vi "ETH 2 Main.vi"(7 "ETH2 Q":refnum<queue>, 8 "error in":errorcluster, 10 "connection ID":refnum<k5>, 11 "data in":string) -> (0 "error out":errorcluster, 2 "connection ID 2":refnum<k5>)   [LabVIEW 2022 SP3]
panel:
  in  "ETH2 Q 2":refnum<queue>
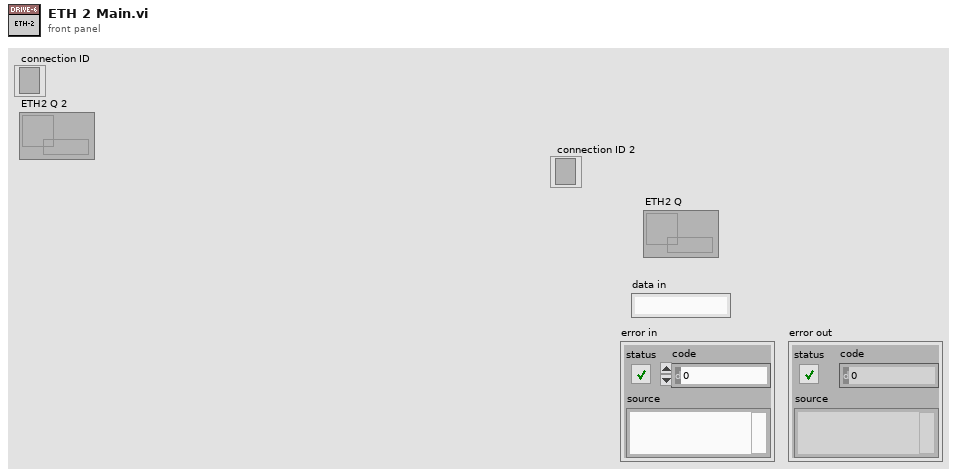
[diagram p1: front panel]
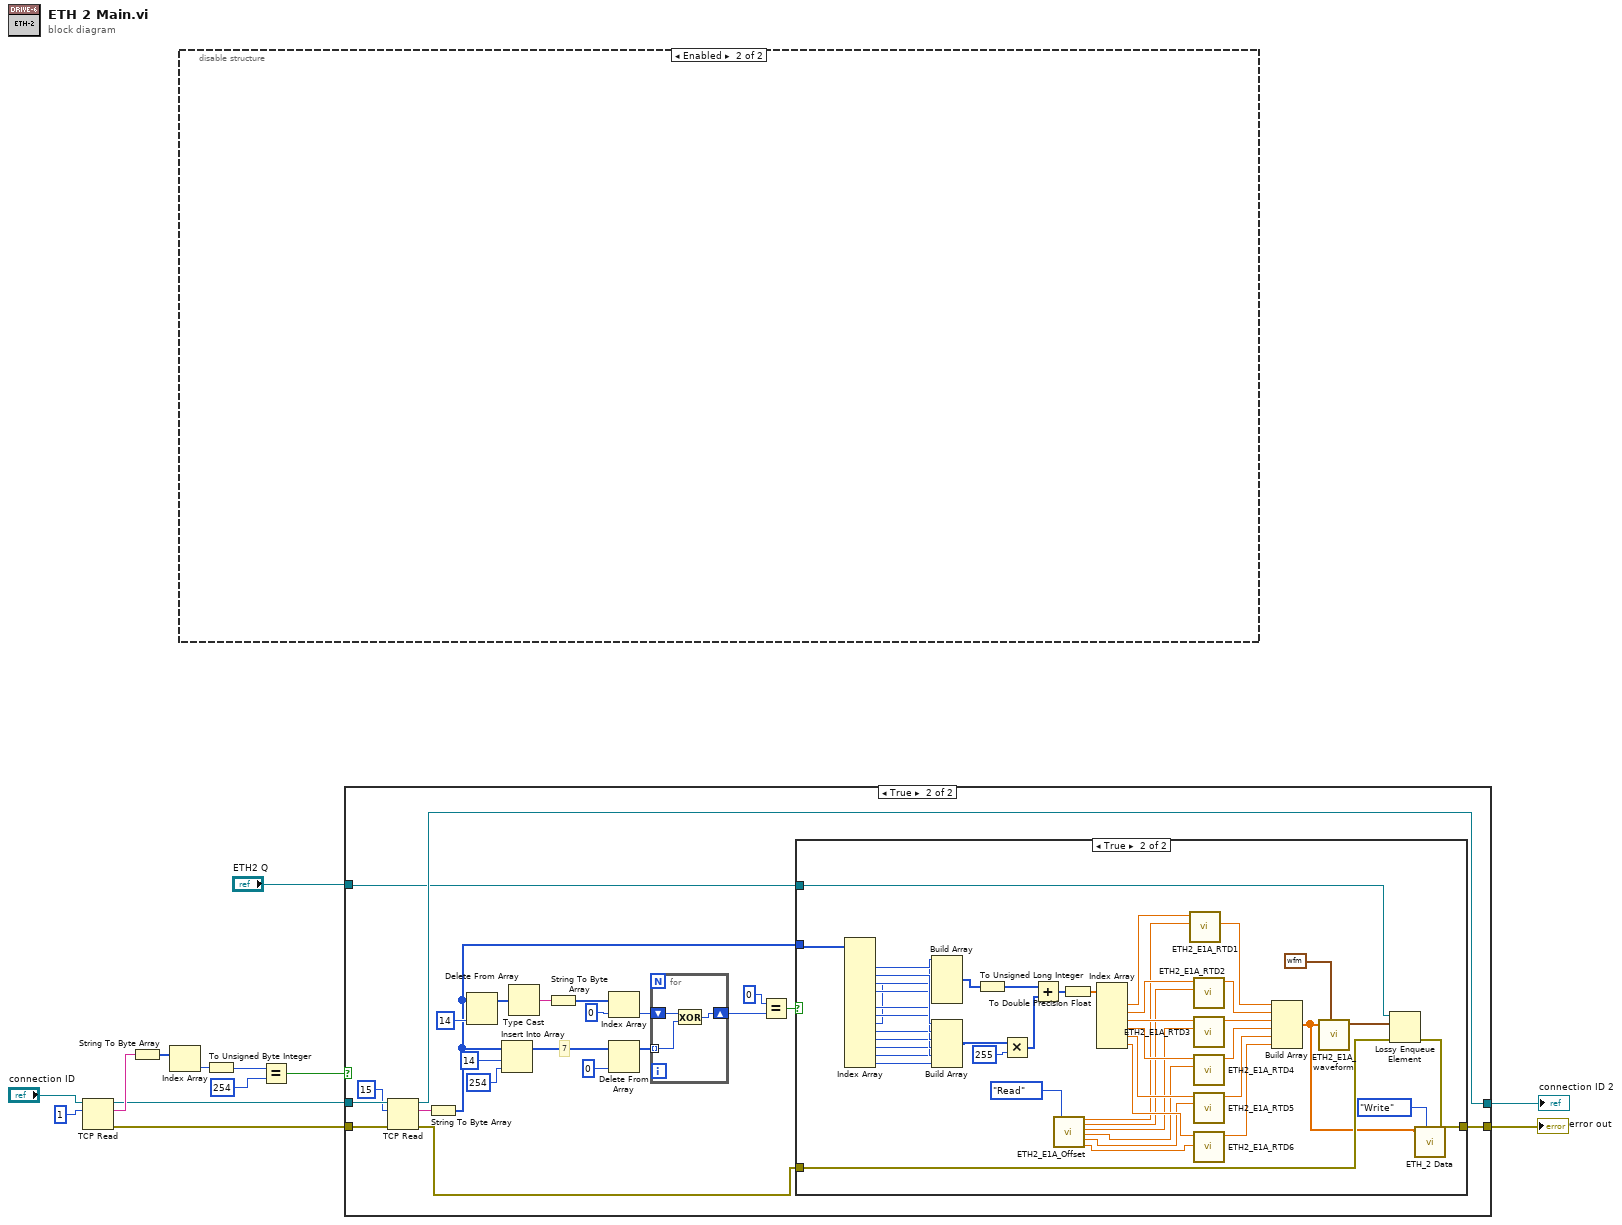
[diagram p0: block diagram]
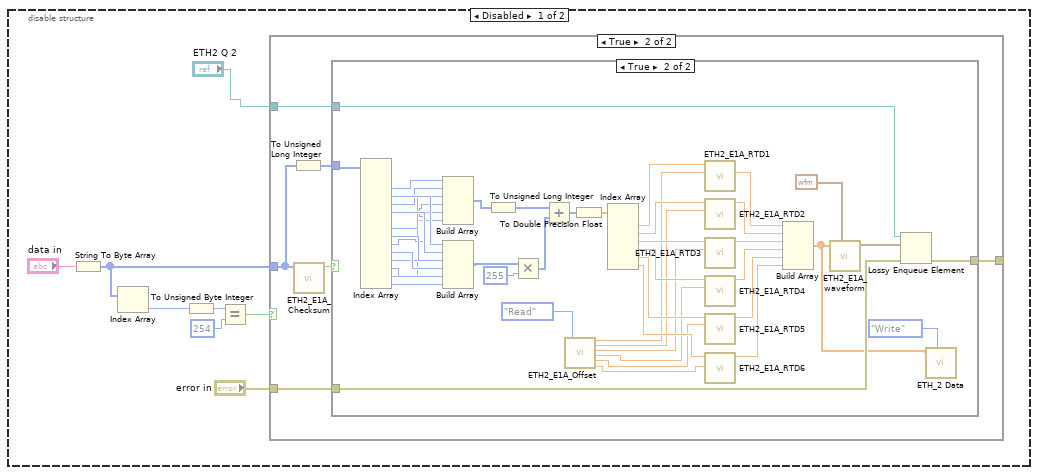
[diagram p2: hidden frame]
diagram:
  n1 = TCP Read(connection ID="connection ID", bytes to read=1) -> (connection ID out=w7:refnum<k5>, data out=w8:string, error out=w5:errorcluster)  [unwired: 3 in]
  n2 = String To Byte Array(string=w8) -> (unsigned byte array=w12:u8[])
  n3 = Index Array(array=w12) -> (element=w11:u8)  [unwired: 1 in]
  n4 = disable-structure shown="Enabled" {
    frame Disabled {
      n5 = String To Byte Array(string="data in") -> (unsigned byte array=w16:u8[])
      n6 = Index Array(array=w16) -> (element=w21:u8)  [unwired: 1 in]
      n7 = To Unsigned Byte Integer(number=w21) -> (unsigned 8bit integer=w20:u8)
      n8 = Equal?(x=w20, y=u8 254) -> (x = y?=w17:bool)
      n9 = case shown="True" w17 {
        tunnel: w16 -> [_ w27]
        tunnel: "ETH2 Q 2" -> [_ w25]
        tunnel: "error in" -> [w22 w24]
        tunnel: [w22 w23] -> _
        frame False {
        }
        frame True {
          n10 = To Unsigned Long Integer(number=w27) -> (unsigned 32bit integer=w26:u32[])
          n11 = call "ETH2_E1A_Checksum.vi"("Data"=w27) -> ("Checksum 2"=w28:bool)  [unwired: 10 in]
          n12 = case shown="True" w28 {
            tunnel: w26 -> [_ w46]
            tunnel: w25 -> [_ w50]
            tunnel: w24 -> [w29 w48]
            tunnel: [w29 w47] -> w23
            frame False {
            }
            frame True {
              n13 = Index Array(array=w46) -> (element #2=w43:u32, element #3=w42:u32, element #4=w41:u32, element #5=w40:u32, element #7=w39:u32, element #8=w38:u32, element #9=w37:u32, element #10=w36:u32, element #11=w35:u32, element #12=w34:u32, element #13=w33:u32, element #14=w32:u32)  [unwired: 14 in, 2 out]
              n14 = Build Array(w43, w41, w39, w37, w35, w33) -> (w45:u32[])
              n15 = Build Array(w42, w40, w38, w36, w34, w32) -> (w44:u32[])
              n16 = To Unsigned Long Integer(number=w45) -> (unsigned 32bit integer=w72:u32[])
              n17 = Multiply(x=w44, y=u32 255) -> (x*y=w74:u32[])
              n18 = Add(x=w72, y=w74) -> (x+y=w71:u32[])
              n19 = call "ETH2_E1A_Offset.vi"("Write/Read"=enum16{"Write", "Read"}."Read") -> ("RTD1 Offset Out"=w63:dbl, "RTD2 Offset Out"=w62:dbl, "RTD3 Offset Out"=w61:dbl, "RTD4 Offset out"=w60:dbl, "RTD5 Offset out"=w59:dbl, "RTD6 Offset  out"=w58:dbl)  [unwired: 13 in]
              n20 = To Double Precision Float(number=w71) -> (double precision float=w75:dbl[])
              n21 = Index Array(array=w75) -> (element #1=w70:dbl, element #2=w69:dbl, element #3=w68:dbl, element #4=w67:dbl, element #5=w66:dbl, element #6=w65:dbl)  [unwired: 6 in]
              n22 = call "ETH2_E1A_RTD1.vi"("RTD 1 Off"=w63, "Input Variable"=w70) -> ("RTD Value"=w57:dbl)  [unwired: 9 in]
              n23 = call "ETH2_E1A_RTD2.vi"("RTD 2 Off"=w62, "Input Variable"=w69) -> ("RTD Value"=w56:dbl)  [unwired: 9 in]
              n24 = call "ETH2_E1A_RTD3.vi"("RTD 3 Off"=w61, "Input Variable"=w68) -> ("RTD Value"=w55:dbl)  [unwired: 9 in]
              n25 = call "ETH2_E1A_RTD4.vi"("RTD 4 Off"=w60, "Input Variable"=w67) -> ("RTD Value"=w54:dbl)  [unwired: 9 in]
              n26 = call "ETH2_E1A_RTD5.vi"("RTD 5 Off"=w59, "Input Variable"=w66) -> ("RTD Value"=w53:dbl)  [unwired: 9 in]
              n27 = call "ETH2_E1A_RTD6.vi"("RTD 6 Off"=w58, "Input Variable"=w65) -> ("RTD Value"=w52:dbl)  [unwired: 9 in]
              n28 = Build Array(w57, w56, w55, w54, w53, w52) -> (w31:dbl[])
              n29 = call "ETH2_E1A_waveform.vi"("Waveform"=waveform(dbl) {"t0"=timestamp(0 s since 1904-01-01), "dt"=0.001, "Y"=[]}, "Array in"=w31) -> ("Array out"=w49:waveform(dbl)[])  [unwired: 9 in]
              n30 = Lossy Enqueue Element(queue=w50, element=w49, error in (no error)=w48) -> (error out=w47:errorcluster)  [unwired: 3 out]
              n31 = call "ETH_2 Data.vi"("Enum"=enum16{"Read", "Write"}."Write", "ETH_2"=w31) -> ()  [unwired: 8 in, 2 out]
            }
          }
        }
      }
    }
    frame Enabled {
    }
  }
  n32 = To Unsigned Byte Integer(number=w11) -> (unsigned 8bit integer=w10:u8)
  n33 = Equal?(x=w10, y=u8 254) -> (x = y?=w6:bool)
  n34 = case shown="True" w6 {
    tunnel: w7 -> [w76 w100]
    tunnel: w5 -> [w77 w99]
    tunnel: [w77 w81] -> w3
    tunnel: [w76 w98] -> w2
    tunnel: "ETH2 Q" -> [_ w78]
    frame False {
    }
    frame True {
      # "7"
      n35 = TCP Read(connection ID=w100, bytes to read=15, error in (no error)=w99) -> (connection ID out=w98:refnum<k5>, data out=w97:string, error out=w80:errorcluster)  [unwired: 2 in]
      n36 = String To Byte Array(string=w97) -> (unsigned byte array=w79:u8[])
      n37 = Delete From Array(array=w79, index=14) -> (array with subset deleted=w88:u8[])  [unwired: 1 in, 1 out]
      n38 = Insert Into Array(array=w79, index=14, new element=u8 254 ("new element/subarray")) -> (w85:u8[])
      n39 = Type Cast(x=w88) -> (*(type *) &x=w94:string)  [unwired: 1 in]
      n40 = String To Byte Array(string=w94) -> (unsigned byte array=w89:u8[])
      n41 = Index Array(array=w89, index=0) -> (element=w92:u8)
      n42 = Delete From Array(array=w85, index=0) -> (array with subset deleted=w91:u8[])  [unwired: 1 in, 1 out]
      n43 = for {
        shift-right: [w149] -> w83
        shift-left: w92 -> [w150]
        tunnel: w91 -> [w148] mode=indexing
        n44 = Exclusive Or(1:w148, 2:w150) -> (0:w149:u8)
      }
      n45 = Equal?(x=u8 0, y=w83) -> (x = y?=w82:bool)
      n46 = case shown="True" w82 {
        tunnel: w79 -> [_ w118]
        tunnel: w78 -> [_ w122]
        tunnel: w80 -> [w101 w120]
        tunnel: [w101 w119] -> w81
        frame False {
        }
        frame True {
          n47 = Index Array(array=w118) -> (element #2=w115:u8, element #3=w114:u8, element #4=w113:u8, element #5=w112:u8, element #7=w111:u8, element #8=w110:u8, element #9=w109:u8, element #10=w108:u8, element #11=w107:u8, element #12=w106:u8, element #13=w105:u8, element #14=w104:u8)  [unwired: 14 in, 2 out]
          n48 = Build Array(w115, w113, w111, w109, w107, w105) -> (w117:u8[])
          n49 = Build Array(w114, w112, w110, w108, w106, w104) -> (w116:u8[])
          n50 = To Unsigned Long Integer(number=w117) -> (unsigned 32bit integer=w144:u32[])
          n51 = Multiply(x=w116, y=u32 255) -> (x*y=w146:u32[])
          n52 = Add(x=w144, y=w146) -> (x+y=w143:u32[])
          n53 = call "ETH2_E1A_Offset.vi"("Write/Read"=enum16{"Write", "Read"}."Read") -> ("RTD1 Offset Out"=w135:dbl, "RTD2 Offset Out"=w134:dbl, "RTD3 Offset Out"=w133:dbl, "RTD4 Offset out"=w132:dbl, "RTD5 Offset out"=w131:dbl, "RTD6 Offset  out"=w130:dbl)  [unwired: 13 in]
          n54 = To Double Precision Float(number=w143) -> (double precision float=w147:dbl[])
          n55 = Index Array(array=w147) -> (element #1=w142:dbl, element #2=w141:dbl, element #3=w140:dbl, element #4=w139:dbl, element #5=w138:dbl, element #6=w137:dbl)  [unwired: 6 in]
          n56 = call "ETH2_E1A_RTD1.vi"("RTD 1 Off"=w135, "Input Variable"=w142) -> ("RTD Value"=w129:dbl)  [unwired: 9 in]
          n57 = call "ETH2_E1A_RTD2.vi"("RTD 2 Off"=w134, "Input Variable"=w141) -> ("RTD Value"=w128:dbl)  [unwired: 9 in]
          n58 = call "ETH2_E1A_RTD3.vi"("RTD 3 Off"=w133, "Input Variable"=w140) -> ("RTD Value"=w127:dbl)  [unwired: 9 in]
          n59 = call "ETH2_E1A_RTD4.vi"("RTD 4 Off"=w132, "Input Variable"=w139) -> ("RTD Value"=w126:dbl)  [unwired: 9 in]
          n60 = call "ETH2_E1A_RTD5.vi"("RTD 5 Off"=w131, "Input Variable"=w138) -> ("RTD Value"=w125:dbl)  [unwired: 9 in]
          n61 = call "ETH2_E1A_RTD6.vi"("RTD 6 Off"=w130, "Input Variable"=w137) -> ("RTD Value"=w124:dbl)  [unwired: 9 in]
          n62 = Build Array(w129, w128, w127, w126, w125, w124) -> (w103:dbl[])
          n63 = call "ETH2_E1A_waveform.vi"("Waveform"=waveform(dbl) {"t0"=timestamp(0 s since 1904-01-01), "dt"=0.001, "Y"=[]}, "Array in"=w103) -> ("Array out"=w121:waveform(dbl)[])  [unwired: 9 in]
          n64 = Lossy Enqueue Element(queue=w122, element=w121, error in (no error)=w120) -> (error out=w119:errorcluster)  [unwired: 3 out]
          n65 = call "ETH_2 Data.vi"("Enum"=enum16{"Read", "Write"}."Write", "ETH_2"=w103) -> ()  [unwired: 8 in, 2 out]
        }
      }
    }
  }
  "error out" <- w3
  "connection ID 2" <- w2
